vi "Read Single File Properties.vi"(8 "error in (no error)":errorcluster, 11 "File Path":path) -> (0 "error out":errorcluster, 2 "File Properties":T1, 3 "File Ref":refnum<vi>)   [LabVIEW 2020, in "DocTool.lvlib"]
uses:
  DocTool.lvlib
  TDefs/Single File Properties.ctl
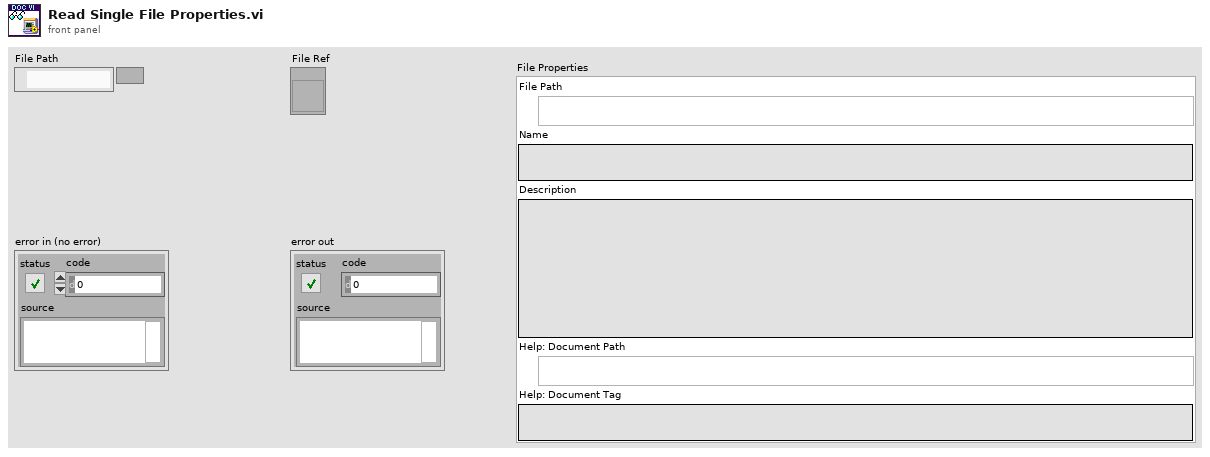
[diagram p1: front panel]
types:
  T1 = typedef "DocTool.lvlib/Single File Properties.ctl" = cluster{"File Path":path, "Name":string, "Description":string, "Help: Document Path":path, "Help: Document Tag":string}
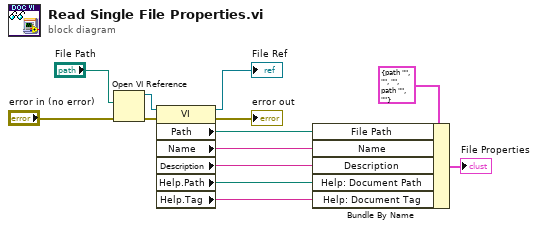
[diagram p0: block diagram]
diagram:
  n1 = Open VI Reference(vi path="File Path", error in (no error)="error in (no error)") -> (vi reference=w7:refnum<vi>, error out=w6:errorcluster)  [unwired: 4 in]
  n2 = property class="VI"(reference=w7, error in=w6) -> (reference out=→"File Ref":refnum<vi>, error out=→"error out":errorcluster, "Path"=w5:path, "Name"=w4:string, "Description"=w3:string, "Help.Path"=w2:path, "Help.Tag"=w1:string)
  n3 = Bundle By Name(cluster=T1 {"File Path"=path "", "Name"="", "Description"="", "Help: Document Path"=path "", "Help: Document Tag"=""} ("File Properties in"), "File Path"=w5, "Name"=w4, "Description"=w3, "Help: Document Path"=w2, "Help: Document Tag"=w1) -> (→"File Properties":T1)
